vi "Replace Element in 2D Array.vi"(6 "format string (%d)":string="%d", 8 "Column":i32, 9 "Value":dbl, 10 "Row":i32, 11 "ItemNames in":string[][](array[string])) -> (3 "ItemNames out":string[][](array[string]))   [LabVIEW 2018, in "EMS User Interface Actor.lvlib" / "EMS User Interface.lvclass"]
uses:
  EMS User Interface.lvclass
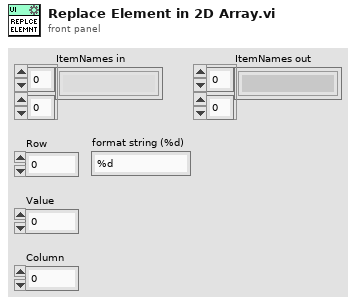
[diagram p1: front panel]
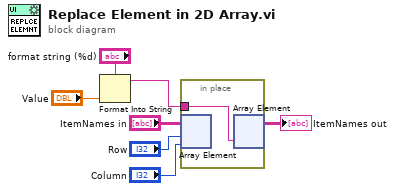
[diagram p0: block diagram]
diagram:
  n1 = Format Into String(format string="format string (%d)", "Value") -> (resulting string=w5:string)  [unwired: 2 in, 1 out]
  n2 = in-place {
    in-place-border: w5 -> [w8]
    n3 = in-place-array #1("ItemNames in", "Row", "Column") -> ()  [unwired: 1 out]
    n4 = in-place-array #1(w8) -> (→"ItemNames out":string[][])  [unwired: 2 out]
  }
